vi "ChildImplementationDefaultValue--Constant.vi"() -> (3 "ChildImplementationDefaultValue":string)   [LabVIEW 2021, in "IconEditorDefaultPlugin.lvlib" / "IconEditorDefaultPlugin.lvclass"]
uses:
  <resource>/plugins/NIIconEditor/UI/Default/IconEditorDefaultPlugin.lvclass
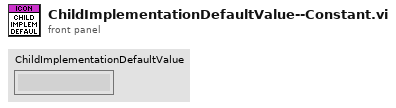
[diagram p1: front panel]
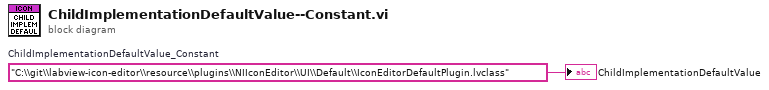
[diagram p0: block diagram]
diagram:
  w1 = "C:\\git\\labview-icon-editor\\resource\\plugins\\NIIconEditor\\UI\\Default\\IconEditorDefaultPlugin.lvclass"  # ChildImplementationDefaultValue_Constant
  "ChildImplementationDefaultValue" <- w1
